vi "APSxIndexPointCalInit.vi"(8 "error in (no error)":errorcluster caption="错误输入（无错误）", 11 "hASIC":i32) -> (0 "error out":errorcluster caption="错误输出")   [LabVIEW 2018]
doc: "该模板用于创建子VI。"
uses:
  APSx.dll/APSx.dll
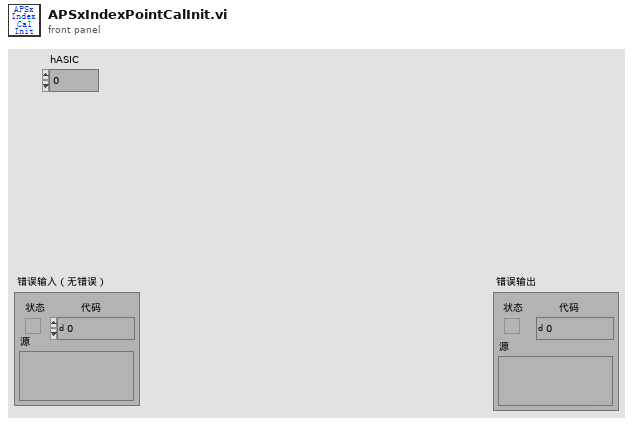
[diagram p1: front panel]
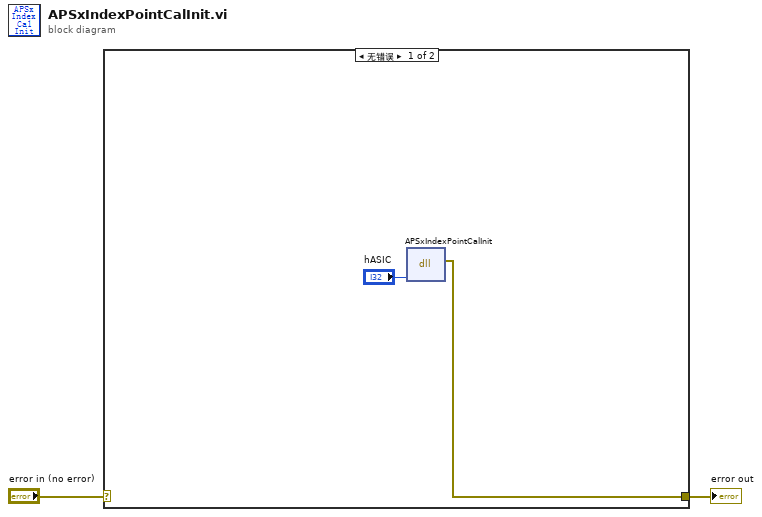
[diagram p0: block diagram]
diagram:
  n1 = case shown="无错误" "error in (no error)" {
    selector: "error in (no error)" -> [_ w5]
    tunnel: [w4 w5] -> w1
    frame No Error {
      n2 = dll-call lib="PTH2]abs D项目Feng恒隆项目Labview传感器对中台SourcesAPSx.dllAPSx.dll" fn="APSxIndexPointCalInit"("hASIC"="hASIC") -> (error out=w4:errorcluster)  [unwired: 5 in, 1 out]
    }
    frame Error {
    }
  }
  "error out" <- w1
